vi "DEMO.vi"() -> ()   [LabVIEW 2013]
uses:
  MallardDuck.lvclass/MallardDuck.lvclass
  WildTurkey.lvclass/WildTurkey.lvclass
  TurkeyAdapter.lvclass/TurkeyAdapter.lvclass
  Duck.lvclass/Duck.lvclass
panel:
  out "野生火雞":string
  out "野生火雞頂替的綠頭鴨 !!":string
  out "真正的綠頭鴨...":string
  # "轉接器模式簡例"
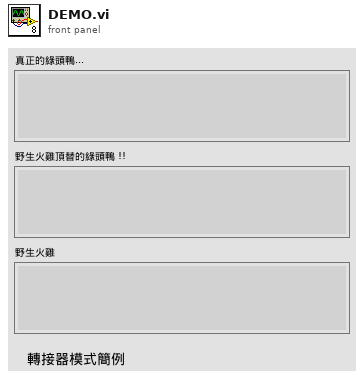
[diagram p1: front panel]
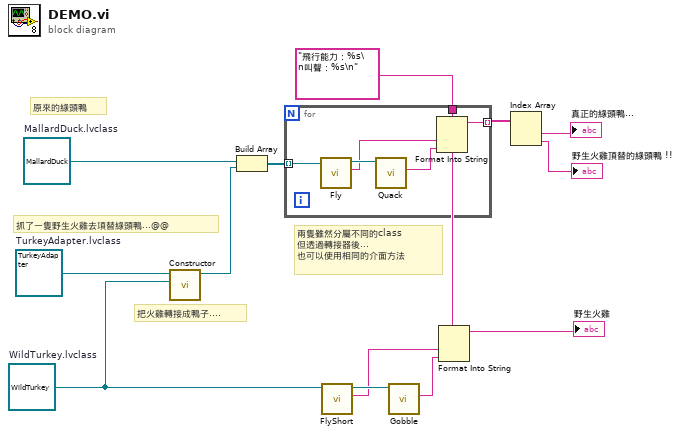
[diagram p0: block diagram]
diagram:
  w2 = "飛行能力：%s\n叫聲：%s\n" ("format string")
  w13 = refnum<class "TurkeyAdapter.lvclass"> refnum  # TurkeyAdapter.lvclass
  w6 = refnum<class "WildTurkey.lvclass"> refnum  # WildTurkey.lvclass
  w12 = refnum<class "MallardDuck.lvclass"> refnum  # MallardDuck.lvclass
  # "兩隻雖然分屬不同的class\n但透過轉接器後...\n也可以使用相同的介面方法"
  # "把火雞轉接成鴨子...."
  # "原來的綠頭鴨"
  # "抓了一隻野生火雞去項替綠頭鴨...@@"
  n1 = call-dynamic "Constructor.vi"("Turkey.lvclass"=w6, "TurkeyAdapter in"=w13) -> ("TurkeyAdapter out"=w11:refnum<class "TurkeyAdapter.lvclass">)  [unwired: 8 in, 1 out]
  n2 = Build Array(w12, w11) -> (w10:refnum<class "Duck.lvclass">[])
  n3 = for {
    tunnel: w10 -> [w18] mode=indexing
    tunnel: [w15] -> w9 mode=indexing
    tunnel: w2 -> [w14]
    n4 = call-dynamic "Fly.vi"("Duck in"=w18) -> ("Fly"=w17:string, "Duck out"=w19:refnum<class "Duck.lvclass">)  [unwired: 8 in, 1 out]
    n5 = call-dynamic "Quack.vi"("Duck in"=w19) -> ("Quack"=w16:string)  [unwired: 8 in, 2 out]
    n6 = Format Into String(format string=w14, w17, w16) -> (resulting string=w15:string)  [unwired: 2 in, 1 out]
  }
  n7 = call-dynamic "FlyShort.vi"("WildTurkey in"=w6) -> ("Fiy"=w4:string, "WildTurkey out"=w5:refnum<class "WildTurkey.lvclass">)  [unwired: 8 in, 1 out]
  n8 = call-dynamic "Gobble.vi"("WildTurkey in"=w5) -> ("Gobble"=w3:string)  [unwired: 8 in, 2 out]
  n9 = Format Into String(format string=w2, w4, w3) -> (resulting string=→"野生火雞":string)  [unwired: 2 in, 1 out]
  n10 = Index Array(array=w9) -> (element #1=→"真正的綠頭鴨...":string, element #2=→"野生火雞頂替的綠頭鴨 !!":string)  [unwired: 2 in]
